vi "_TangoSubscribeAttributePeriodicEvent.vi"(1 "error in":errorcluster, 2 "attribute name":string, 3 "device name":string, 4 "attribute event ref.":T1) -> (0 "error out":errorcluster)   [LabVIEW 2014, in "tango.lvlib"]
uses:
  tango.lvlib
  Common VIs/Typedefs/_AttributeEventRef.ctl
  Common VIs/Typedefs/_AttributeValue_t.ctl
  Common VIs/Typedefs/_AttributeQuality_t.ctl
  Common VIs/Typedefs/_AttributeDataType_t.ctl
  _EventType.ctl
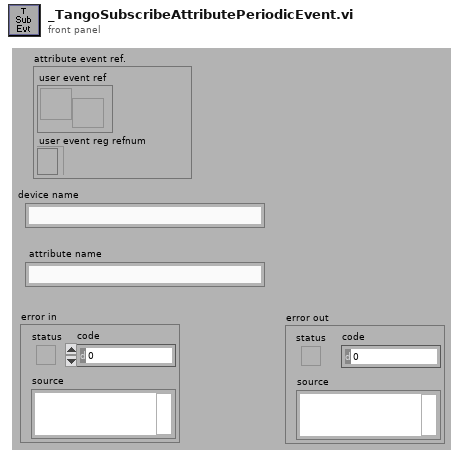
[diagram p1: front panel]
types:
  T1 = typedef "tango.lvlib/_AttributeEventRef.ctl" = cluster{"user event ref":refnum<user-event>, "user event reg refnum":refnum<event-registration>}
  T2 = typedef "tango.lvlib/_EventType.ctl" = enum32{"CHANGE_EVENT", "DEPRECATED_QUALITY_EVENT", "PERIODIC_EVENT", "ARCHIVE_EVENT", "USER_EVENT", "ATTRIBUTE_CONF_EVENT", "DATA_READY_EVENT", "INTERFACE_CHANGE_EVENT", "UNKNOWN_EVENT"}
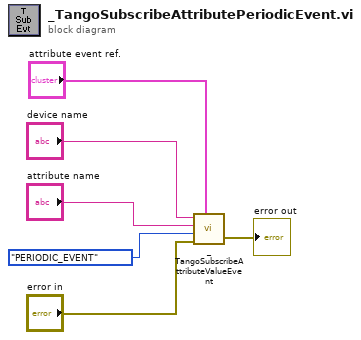
[diagram p0: block diagram]
diagram:
  n1 = call "_TangoSubscribeAttributeValueEvent.vi"("device name"="device name", "attribute name"="attribute name", "tango event type"=_EventType."PERIODIC_EVENT", "error in"="error in", "attribute event ref."="attribute event ref.") -> ("error out"=→"error out":errorcluster)  [unwired: 1 out]
